vi "Handle Errors and Warning.vi"(4 "Error Code":i32 format="%0.0f") -> (1 "Error Out":errorcluster)   [LabVIEW 2014]
uses:
  <vilib>/Utility/error.llb/DialogType.ctl
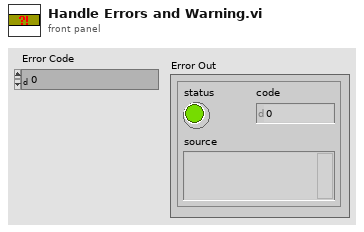
[diagram p1: front panel]
types:
  T1 = typedef "DialogType.ctl" = u16
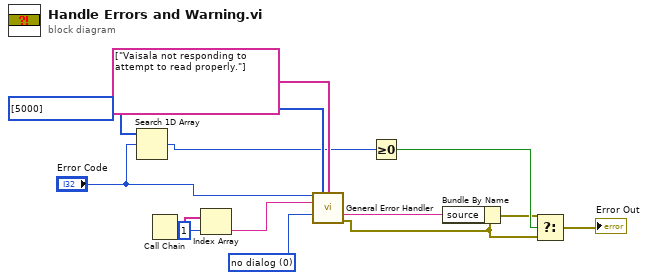
[diagram p0: block diagram]
diagram:
  w13 = T1 0 items=["no dialog", "OK message", "continue or stop message", "OK message + warnings", "continue/stop + warnings"] ("type of dialog (OK msg:1)")
  w9 = i32[] [5000] ("[user-defined codes]")
  n1 = Search 1D Array(1D array=w9, element="Error Code") -> (index of element=w6:i32)  [unwired: 1 in]
  n2 = Call Chain() -> (call chain=w12:string[])
  n3 = Index Array(array=w12, index=1) -> (element=w10:string)
  n4 = call <vilib>:"General Error Handler.vi"("[error code] (0)"="Error Code", "[user-defined codes]"=w9, "[user-defined descriptions]"=string[] ["Vaisala not responding to attempt to read properly."], "[error source] (\" \")"=w10, "type of dialog (OK msg:1)"=w13) -> ("message"=w5:string, "error out"=w2:errorcluster)  [unwired: 6 in, 3 out]
  n5 = Greater Or Equal To 0?(x=w6) -> (x >= 0?=w4:bool)
  n6 = Bundle By Name(cluster=w2, "source"=w5) -> (w3:errorcluster)
  n7 = Select(t=w3, s=w4, f=w2) -> (s? t:f=→"Error Out":errorcluster)
